vi "Copy Reports to server.vi"(9 "Path to copy to?":path=path "E:/UGDGNEW/17.05.2013-12.59", 11 "Path to copy from?":path=path "C:/Windows/Temp/New folder") -> ()   [LabVIEW 2012]
panel:
  out "Array":path[](array[path])
  out "All Files in Dir":path[](array[path])
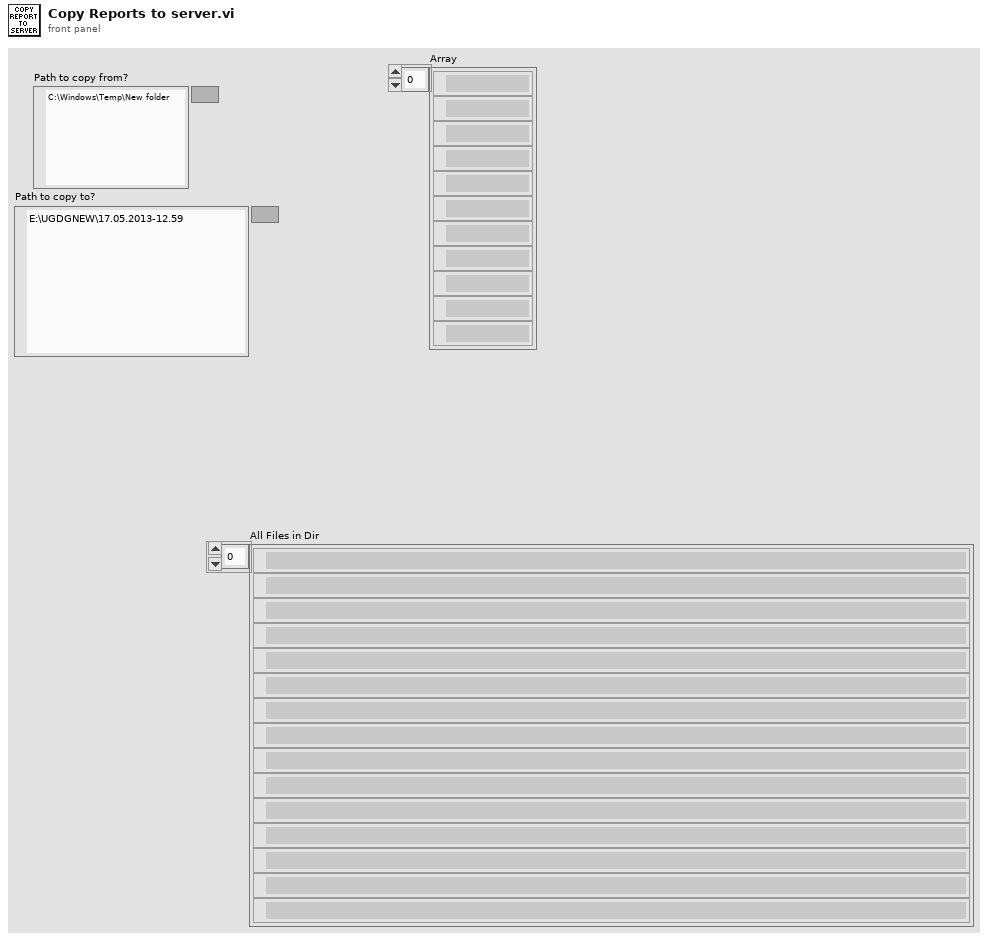
[diagram p1: front panel]
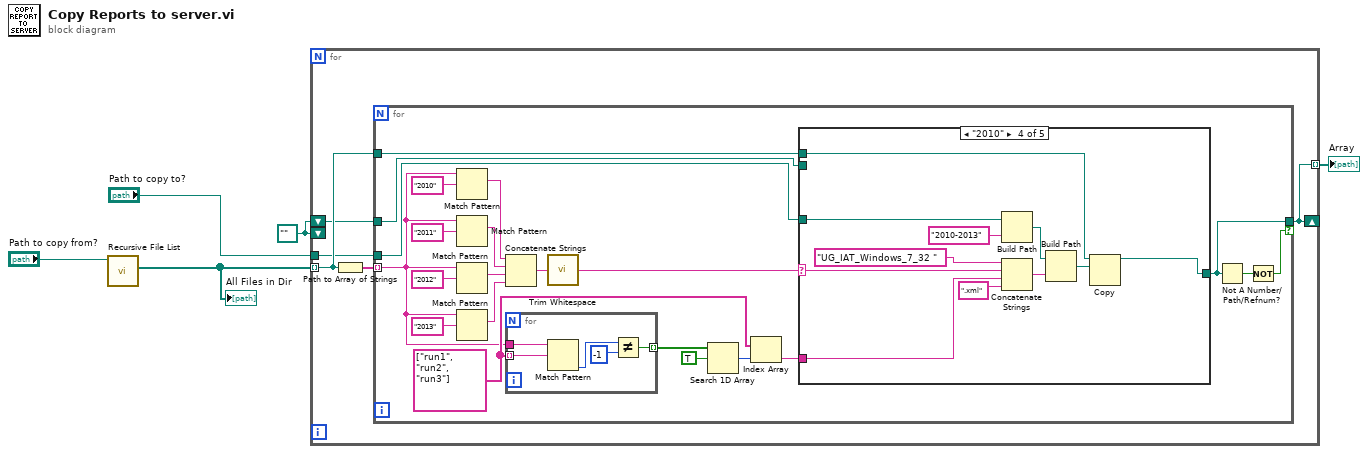
[diagram p0: block diagram]
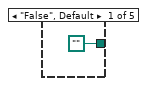
[diagram p2: hidden frame]
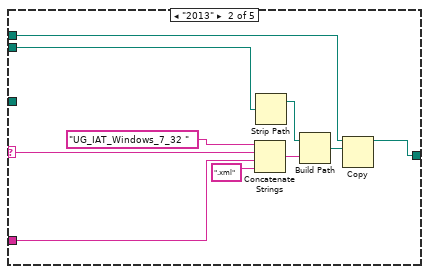
[diagram p3: hidden frame]
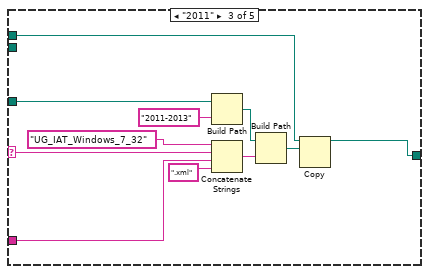
[diagram p4: hidden frame]
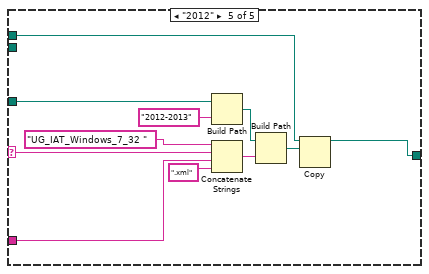
[diagram p5: hidden frame]
diagram:
  w2 = path "" ("new path")
  n1 = call <vilib>:"Recursive File List.vi"("Folder Path"="Path to copy from?") -> ("All Files in Dir"=w4:path[])  [unwired: 6 in, 4 out]
  "All Files in Dir" <- w4
  n2 = for {
    tunnel: w4 -> [w9] mode=indexing
    tunnel: "Path to copy to?" -> [w8]
    shift-right: [w6] -> _
    shift-left: w2 -> [w7]
    shift-left: w2 -> [_]
    tunnel: [w6] -> w1 mode=indexing
    n3 = Path to Array of Strings(0:w9) -> (2:w10:string[])  [unwired: 1 out]
    n4 = for {
      tunnel: w10 -> [w14] mode=indexing
      tunnel: w9 -> [w32]
      tunnel: w8 -> [w31]
      tunnel: w7 -> [w17]
      tunnel: [w11] -> w6 if=w15
      w28 = string[] ["run1", "run2", "run3"]
      n5 = Match Pattern(string=w14, regular expression="2010") -> (match substring=w21:string)  [unwired: 1 in, 3 out]
      n6 = Match Pattern(string=w14, regular expression="2011") -> (match substring=w20:string)  [unwired: 1 in, 3 out]
      n7 = Match Pattern(string=w14, regular expression="2012") -> (match substring=w19:string)  [unwired: 1 in, 3 out]
      n8 = Match Pattern(string=w14, regular expression="2013") -> (match substring=w12:string)  [unwired: 1 in, 3 out]
      n9 = Concatenate Strings(w21, w20, w19, w12) -> (w18:string)
      n10 = for {
        tunnel: w14 -> [w81]
        tunnel: w28 -> [w80] mode=indexing
        tunnel: [w77] -> w29 mode=indexing
        n11 = Match Pattern(string=w81, regular expression=w80) -> (offset past match=w78:i32)  [unwired: 1 in, 3 out]
        n12 = Not Equal?(x=w78, y=-1) -> (x != y?=w77:bool)
      }
      n13 = call <vilib>:"Trim Whitespace.vi"("string"=w18) -> ("trimmed string"=w24:string)  [unwired: 1 in]
      n14 = Search 1D Array(1D array=w29, element=TRUE) -> (index of element=w27:i32)  [unwired: 1 in]
      n15 = Index Array(array=w28, index=w27) -> (element=w26:string)
      n16 = case shown="\"2010\"" w24 {
        selector: w24 -> [_ w37 w49 w60 w71]
        tunnel: w32 -> [_ w42 w54 w65 w76]
        tunnel: w31 -> [_ _ w53 w64 w75]
        tunnel: w26 -> [_ w36 w50 w61 w72]
        tunnel: [path "" w34 w44 w55 w66] -> w11
        tunnel: w17 -> [_ w43 _ _ _]
        frame "False", Default {
        }
        frame "2013" {
          n17 = Concatenate Strings("UG_IAT_Windows_7_32 " ("string"), w37, w36, ".xml" ("string")) -> (w35:string)
          n18 = Strip Path(path=w43) -> (stripped path=w40:path)  [unwired: 1 out]
          n19 = Build Path(base path=w40, name or relative path=w35) -> (appended path=w41:path)
          n20 = Copy(10:w41, 11:w42) -> (3:w34:path)  [unwired: 3 in, 2 out]
        }
        frame "2011" {
          n21 = Build Path(base path=w53, name or relative path="2011-2013") -> (appended path=w47:path)
          n22 = Concatenate Strings("UG_IAT_Windows_7_32" ("string"), w49, w50, ".xml" ("string")) -> (w46:string)
          n23 = Build Path(base path=w47, name or relative path=w46) -> (appended path=w45:path)
          n24 = Copy(10:w45, 11:w54) -> (3:w44:path)  [unwired: 3 in, 2 out]
        }
        frame "2010" {
          n25 = Build Path(base path=w64, name or relative path="2010-2013") -> (appended path=w58:path)
          n26 = Concatenate Strings("UG_IAT_Windows_7_32 " ("string"), w60, w61, ".xml" ("string")) -> (w57:string)
          n27 = Build Path(base path=w58, name or relative path=w57) -> (appended path=w56:path)
          n28 = Copy(10:w56, 11:w65) -> (3:w55:path)  [unwired: 3 in, 2 out]
        }
        frame "2012" {
          n29 = Build Path(base path=w75, name or relative path="2012-2013") -> (appended path=w69:path)
          n30 = Concatenate Strings("UG_IAT_Windows_7_32 " ("string"), w71, w72, ".xml" ("string")) -> (w68:string)
          n31 = Build Path(base path=w69, name or relative path=w68) -> (appended path=w67:path)
          n32 = Copy(10:w67, 11:w76) -> (3:w66:path)  [unwired: 3 in, 2 out]
        }
      }
      n33 = Not A Number/Path/Refnum?(number/path/refnum=w11) -> (NaN/Path/Refnum?=w16:bool)
      n34 = Not(x=w16) -> (.not. x?=w15:bool)
    }
  }
  "Array" <- w1
